vi "Read scrolling mode.vi"(8 "error in (no error)":errorcluster, 11 "D_Datagrid in":refnum<class "D_Datagrid.lvclass">) -> (0 "error out":errorcluster, 2 "Scrolling mode":T1, 3 "D_Datagrid out":refnum<class "D_Datagrid.lvclass">)   [LabVIEW 2023, in "D Datagrid Library.lvlib" / "D_Datagrid.lvclass"]
uses:
  D_Datagrid.lvclass
  D_Datagrid.lvclass/D_Datagrid.ctl
  Scrolling behavior.ctl
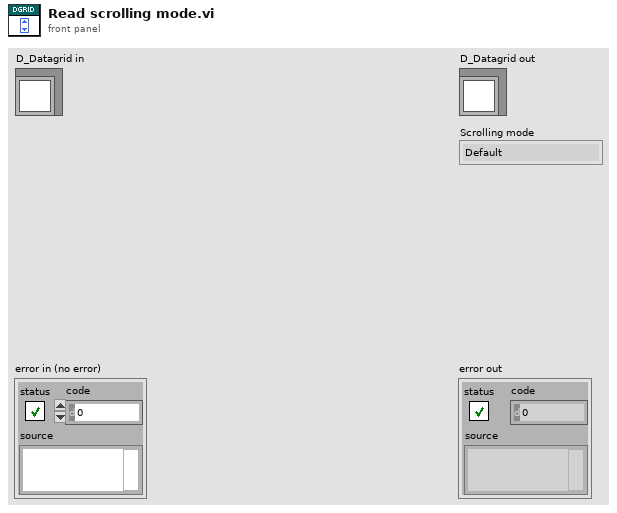
[diagram p1: front panel]
types:
  T1 = typedef "D Datagrid Library.lvlib/D_Datagrid.lvclass/Scrolling behavior.ctl" = enum16{"Default", "Locked", "Displayed items only"}
  T2 = typedef "D Datagrid Library.lvlib/D_Datagrid.lvclass/State Data.ctl" = cluster{"Data elements":refnum<class "DatagridElement.lvclass">[][], "Auto-update indicator":bool, "Scrolling mode":T1}
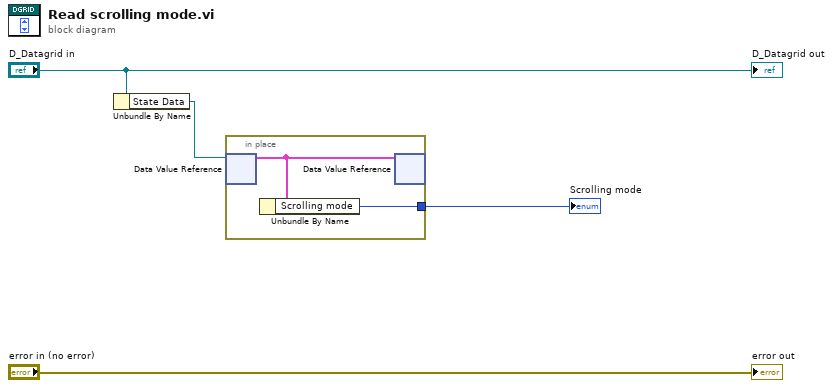
[diagram p0: block diagram]
diagram:
  n1 = Unbundle By Name("D_Datagrid in") -> ("State Data"=w2:refnum<data-value>)
  n2 = in-place {
    in-place-border: [w5] -> w1
    n3 = in-place-dvr #1(w2) -> (w6:T2)  [unwired: 1 out]
    n4 = Unbundle By Name(w6) -> ("Scrolling mode"=w5:T1)
    n5 = in-place-dvr #1(w6) -> ()  [unwired: 2 out]
  }
  "Scrolling mode" <- w1
  "error out" <- "error in (no error)"
  "D_Datagrid out" <- "D_Datagrid in"
